vi "AssertValueByFocusName.vi"(0 "VI Reference In":refnum<vi>, 1 "Test Label":string, 2 "delimiter (>>)":string=">>", 3 "Assert Only? (F)":bool, 5 "Control Path":string, 7 "Item Name":string, 11 "Error In":errorcluster, 12 "Assert Interval(10 ms)":u32=10, 13 "Timeout(5 sec)":dbl=5.0) -> (4 "VI Reference Out":refnum<vi>, 6 "Asserted Value":string, 15 "Error Out":errorcluster)   [LabVIEW 2016, in "Drona.lvlib" / "AssertControlValue.lvlib" / "AssertMCListbox.lvlib"]
doc: "Asserts if the focus item first column name on multi-column listbox controls is equal.\n\nThe input control name is given as a string, incase of the path, use delimiters in between the path.\nThis VI gets the control value until the value is equal to the input value."
uses:
  AssertMCListbox.lvlib
  Get/GetControlRef/GetControlRefByPath.vi
  <vilib>/Utility/error.llb/Error Cluster From Error Code.vi
  <vilib>/addons/_JKI Toolkits/Caraya/classes/Assert/Assert Equal Value_Variant.vi
  <vilib>/ErrorRing/Error Ring.xnode
  <vilib>/addons/_JKI Toolkits/Caraya/classes/Assert/Assert.lvclass
  Get/GetControlRef/GetControlRef.lvlib
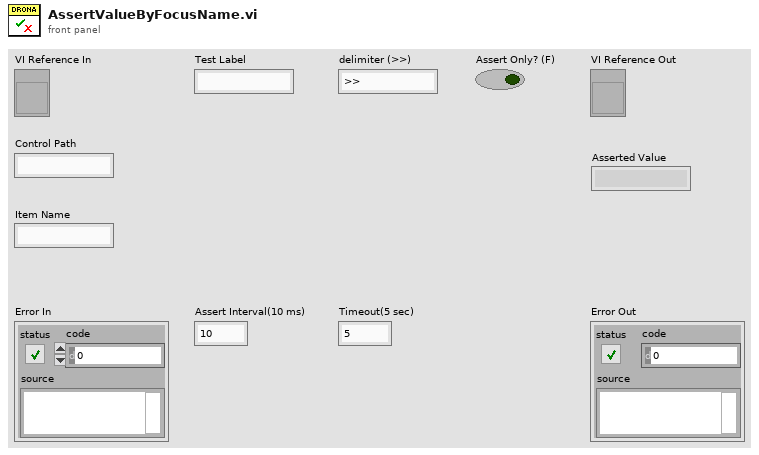
[diagram p1: front panel]
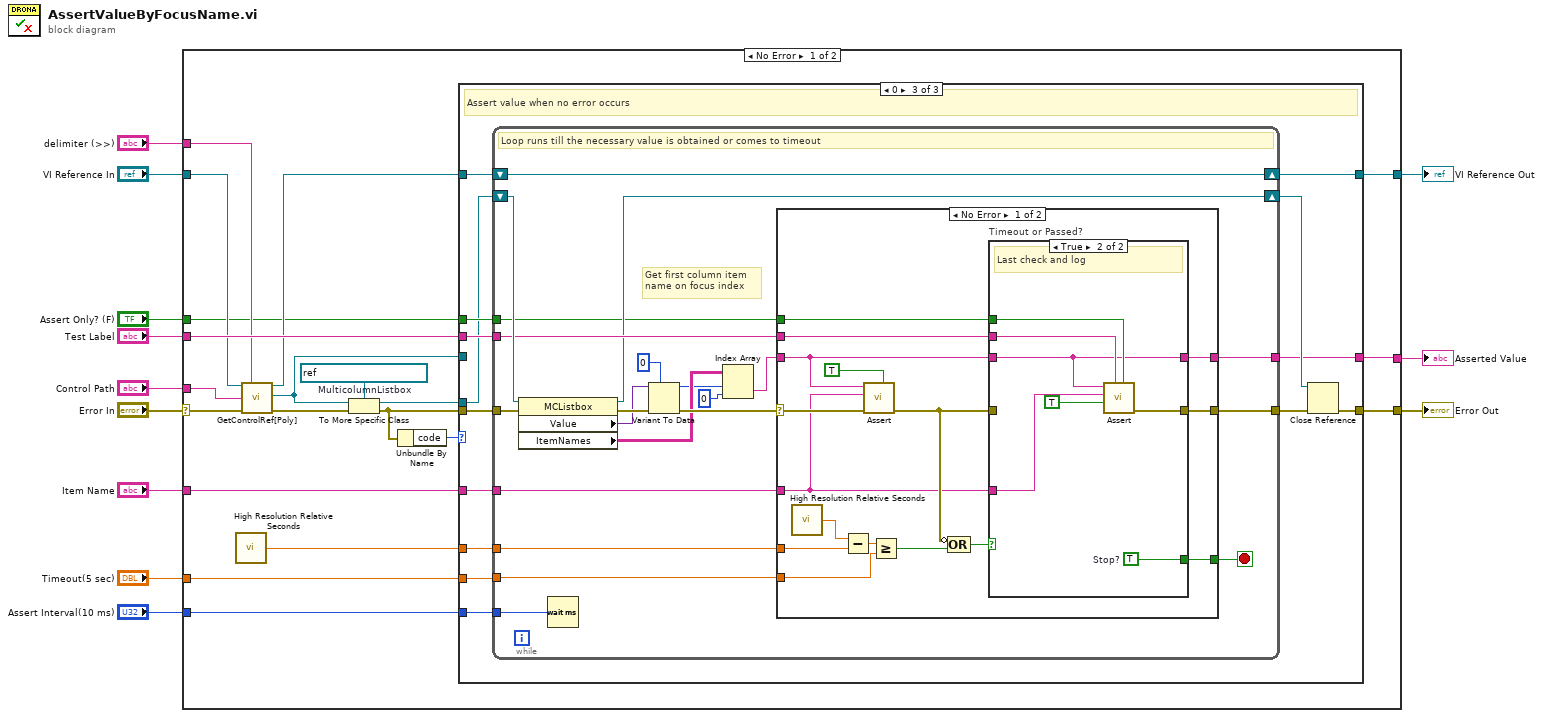
[diagram p0: block diagram]
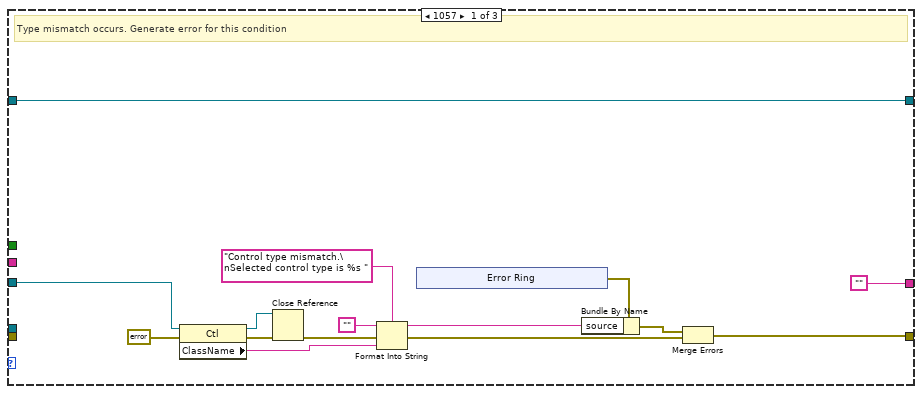
[diagram p2: hidden frame]
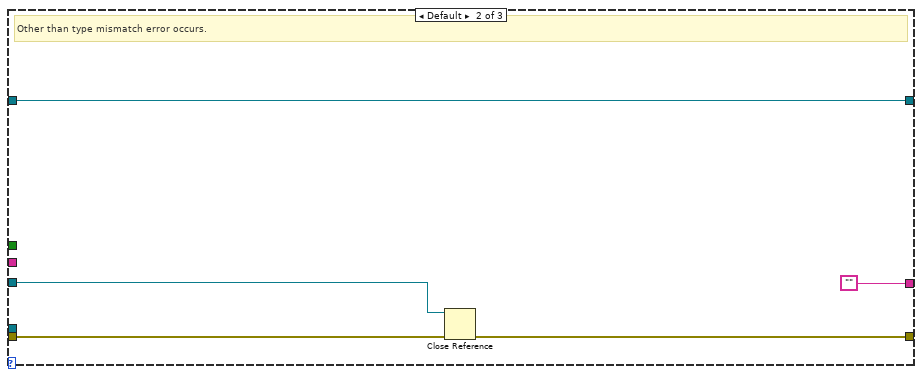
[diagram p3: hidden frame]
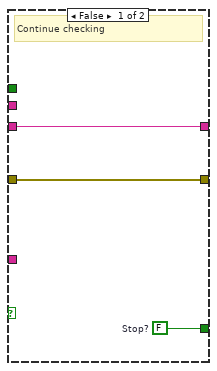
[diagram p4: hidden frame]
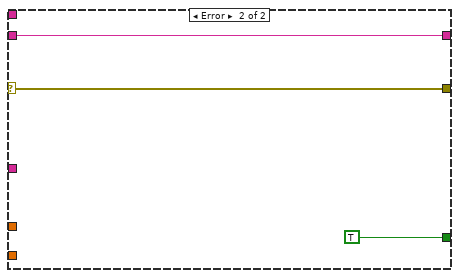
[diagram p5: hidden frame]
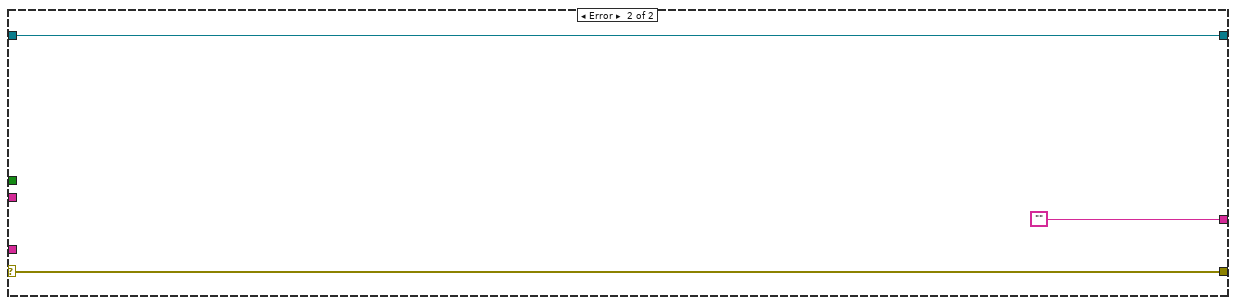
[diagram p6: hidden frame]
diagram:
  n1 = case shown="No Error" "Error In" {
    selector: "Error In" -> [w27 w124]
    tunnel: "Timeout(5 sec)" -> [w32 _]
    tunnel: [w31 w123] -> w11
    tunnel: "Item Name" -> [w30 _]
    tunnel: [w21 w124] -> w10
    tunnel: "Assert Interval(10 ms)" -> [w29 _]
    tunnel: "Test Label" -> [w28 _]
    tunnel: "VI Reference In" -> [w26 w123]
    tunnel: "Control Path" -> [w25 _]
    tunnel: "delimiter (>>)" -> [w20 _]
    tunnel: "Assert Only? (F)" -> [w19 _]
    tunnel: [w18 ""] -> w1
    frame No Error {
      w17 = refnum<vi> refnum  # MulticolumnListbox
      n2 = call <vilib>:"High Resolution Relative Seconds.vi"() -> ("relative seconds"=w24:dbl)
      n3 = call-poly "GetControlRef[Poly].vi"("VI Reference In"=w26, "delimiter (>>)"=w20, "Control Path"=w25, "error In"=w27) -> ("VI Reference Out"=w22:refnum<vi>, "Ctl Refnum"=w13:refnum<vi>, "error out"=w23:errorcluster)  [unwired: 9 in]
      n4 = To More Specific Class(target class=w17, reference=w13, error in=w23) -> (specific class reference=w16:refnum<vi>, error out=w15:errorcluster)
      n5 = Unbundle By Name(w15) -> ("code"=w14:i32)
      n6 = case shown="0" w14 {
        tunnel: w32 -> [_ _ w71]
        tunnel: [w47 w57 w70] -> w31
        tunnel: w30 -> [_ _ w69]
        tunnel: w29 -> [_ _ w67]
        tunnel: w28 -> [_ _ w66]
        tunnel: w24 -> [_ _ w65]
        tunnel: w22 -> [w47 w57 w64]
        tunnel: [w34 w54 w63] -> w21
        tunnel: w19 -> [_ _ w61]
        tunnel: ["" "" w60] -> w18
        tunnel: w15 -> [_ w56 w59]
        tunnel: w16 -> [_ _ w58]
        tunnel: w13 -> [w33 w53 _]
        frame 1057 {
          # "Type mismatch occurs. Generate error for this condition"
          n7 = property class="Ctl"(reference=w33, error in=errorcluster {"status"=FALSE, "code"=0, "source"=""} ("error out")) -> (reference out=w35:refnum<vi>, error out=w45:errorcluster, "ClassName"=w42:string)
          n8 = Close Reference(reference=w35, error in (no error)=w45) -> (error out=w36:errorcluster)
          n9 = Format Into String(format string="Control type mismatch.\nSelected control type is %s ", initial string="", error in=w36, w42) -> (resulting string=w39:string, error out=w37:errorcluster)
          n10 = xnode "Error Ring"() -> ("error out"=w40:errorcluster)
          n11 = Bundle By Name(cluster=w40, "source"=w39) -> (w38:errorcluster)
          n12 = Merge Errors(w38, w37) -> (w34:errorcluster)
        }
        frame Default {
          # "Other than type mismatch error occurs."
          n13 = Close Reference(reference=w53, error in (no error)=w56) -> (error out=w54:errorcluster)
        }
        frame 0 {
          # "Assert value when no error occurs"
          n14 = while {
            tunnel: w69 -> [w79]
            tunnel: w71 -> [w91]
            tunnel: w65 -> [w92]
            tunnel: w59 -> [w86]
            tunnel: [w89] -> w68
            tunnel: w67 -> [w87]
            tunnel: w66 -> [w83]
            shift-right: [w84] -> w70
            shift-left: w64 -> [w84]
            shift-right: [w82] -> w62
            shift-left: w58 -> [w85]
            tunnel: w61 -> [w81]
            tunnel: [w80] -> w60
            stop <- w90 stop-if-true
            # "Get first column item \nname on focus index"
            # "Loop runs till the necessary value is obtained or comes to timeout"
            n15 = property on="Property Node" class="MCListbox"(reference=w85, error in=w86) -> (reference out=w82:refnum<vi>, error out=w88:errorcluster, "Value"=w77:variant, "ItemNames"=w75:string[][])
            n16 = Wait (ms)(milliseconds to wait=w87) -> ()  [unwired: 1 out]
            n17 = Variant To Data(error in=w88, type=0, Variant=w77) -> (data=w73:i32, error out=w78:errorcluster)
            n18 = Index Array(array=w75, index (row)=w73, index (col)=0 ("disabled index (col)")) -> (element=w72:string)
            n19 = case shown="No Error" w78 {
              selector: w78 -> [w104 w121]
              tunnel: w92 -> [w108 _]
              tunnel: w91 -> [w105 _]
              tunnel: [w95 TRUE] -> w90
              tunnel: [w96 w121] -> w89
              tunnel: w79 -> [w97 _]
              tunnel: w72 -> [w98 w119]
              tunnel: w83 -> [w103 _]
              tunnel: w81 -> [w94 _]
              tunnel: [w93 w119] -> w80
              frame No Error {
                n20 = call <vilib>:"High Resolution Relative Seconds.vi"() -> ("relative seconds"=w107:dbl)
                n21 = Subtract(x=w107, y=w108) -> (x-y=w106:dbl)
                n22 = call-poly <vilib>:"Assert.vi"("Assert Only? (F)"=TRUE, "error in (no error)"=w104, "Y"=w97, "X"=w98) -> ("error out"=w101:errorcluster)  [unwired: 6 in, 1 out]
                n23 = Greater Or Equal?(x=w106, y=w105) -> (x >= y?=w102:bool)
                n24 = Compound Arithmetic op=OR(invert w101, w102) -> (w100:bool)
                n25 = case "Timeout or Passed?" shown="True" w100 {
                  tunnel: w101 -> [w111 _]
                  tunnel: w97 -> [_ w114]
                  tunnel: w98 -> [w109 w113]
                  tunnel: w103 -> [_ w118]
                  tunnel: [w111 w117] -> w96
                  tunnel: [w110 w116] -> w95
                  tunnel: w94 -> [_ w115]
                  tunnel: [w109 w113] -> w93
                  frame False {
                    w110 = FALSE  # Stop?
                    # "Continue checking"
                  }
                  frame True {
                    w116 = TRUE  # Stop?
                    # "Last check and log"
                    n26 = call-poly <vilib>:"Assert.vi"("Assert Only? (F)"=w115, "Label"=w118, "Register with caller test (F)"=TRUE, "Y"=w114, "X"=w113) -> ("error out"=w117:errorcluster)  [unwired: 5 in, 1 out]
                  }
                }
              }
              frame Error {
              }
            }
          }
          n27 = Close Reference(reference=w62, error in (no error)=w68) -> (error out=w63:errorcluster)
        }
      }
    }
    frame Error {
    }
  }
  "Error Out" <- w10
  "VI Reference Out" <- w11
  "Asserted Value" <- w1
